vi "calc_focus.vi"(8 "error in":errorcluster, 10 "Image":T1) -> (0 "error out":errorcluster, 2 "focus":sgl, 3 "return value":i32)   [LabVIEW 2017, in "Vision.lvlib"]
uses:
  Vision.lvlib
  bin/Vision.dll
  <vilib>/vision/Image Controls.llb/IMAQ Image.ctl
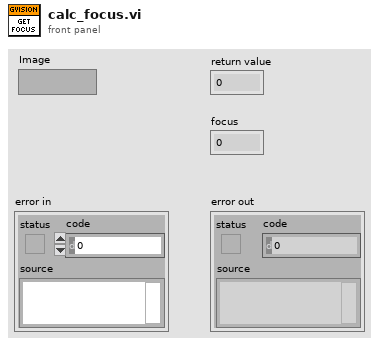
[diagram p1: front panel]
types:
  T1 = typedef "IMAQ Image.ctl" = refnum<image>
  T2 = enum32{"Map Pixel Pointer", "Unmap Pixel Pointer", "Get Pixels Infos"}
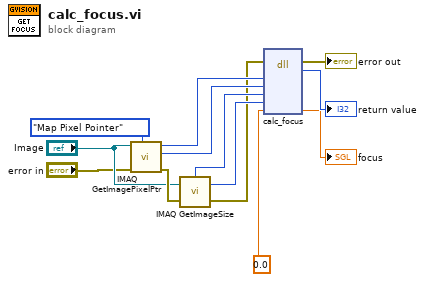
[diagram p0: block diagram]
diagram:
  n1 = call "IMAQ GetImagePixelPtr"("Function"=T2."Map Pixel Pointer", "error in (no error)"="error in", "Image"="Image") -> ("error out"=w8:errorcluster, "LineWidth(Pixels)"=w5:i32, "Pixel Pointer out"=w6:u64)  [unwired: 3 in, 3 out]
  n2 = call "IMAQ GetImageSize"("Image"="Image", "error in (no error)"=w8) -> ("Y Resolution"=w3:i32, "X Resolution"=w4:i32, "error out"=w1:errorcluster)  [unwired: 2 in]
  n3 = dll-call lib="C:/Users/Caleb/Desktop/nebraska-silicon-lab/pixel-gantry-extra/LV/bin/Vision.dll" fn="calc_focus"(error in=w1, "img"=w6, "imgLineWidth"=w5, "imgWidth"=w4, "imgHeight"=w3, "focus"=sgl 0.0) -> (error out=→"error out":errorcluster, "return type"=→"return value":i32, "focus"=→"focus":sgl)  [unwired: 6 in, 1 out]
